vi "Test.vi"() -> ()   [LabVIEW 2012]
uses:
  Hover Button.xctl
  Button Colors.ctl
  Font Properties.ctl
panel:
  in  "Font":T1
  out "Error Out":errorcluster
  in  "Error In":errorcluster
  in  "Show Boolean Text":bool
  in  "Multiple Strings":bool
  in  "Hover Color":T2={"On Color"=16776960, "Text Color"=0, "Off Color"=16776960}
  in  "Button Color":T2={"On Color"=16860, "Text Color"=16777226, "Off Color"=16860}
  in  "Boolean Text":string[](array[string])=["Off", "Off"]
  in  "stop":bool
  in  "Hover Button":bool(xcontrol)
  # "This is a test vi for the Hover Button Xcontrol.  You should be able\nto click the right button selection menu to change the Hover Button\nProperties.  The controls on the right of the Hover Button show the\nuse of the property nodes defined for the Hover Button."
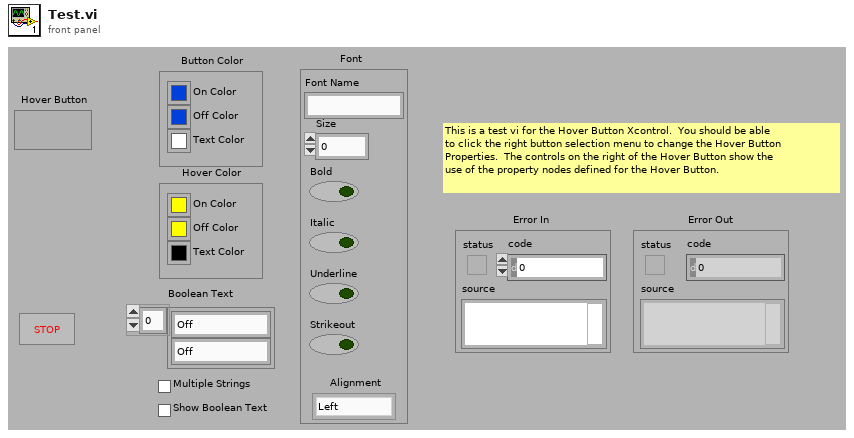
[diagram p1: front panel]
types:
  T1 = typedef "Hover Button.xctl/Font Properties.ctl" = cluster{"Font Name":string, "Size":u32, "Bold":bool, "Italic":bool, "Underline":bool, "Strikeout":bool, "Alignment":enum16{"Left", "Center", "Right"}}
  T2 = typedef "Hover Button.xctl/Button Colors.ctl" = cluster{"On Color":u32, "Text Color":u32, "Off Color":u32}
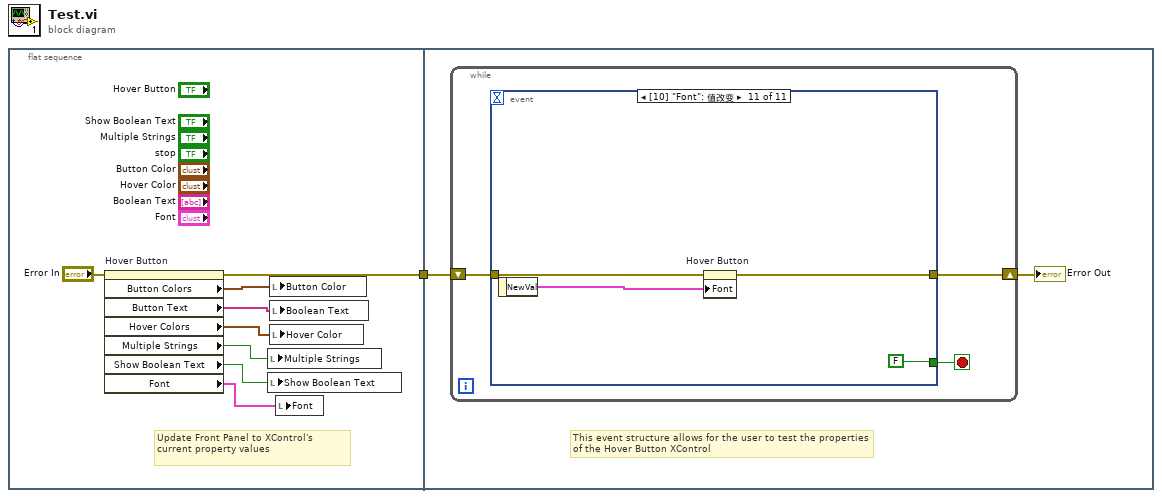
[diagram p0: block diagram]
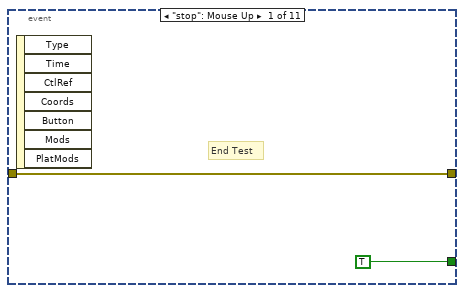
[diagram p2: hidden frame]
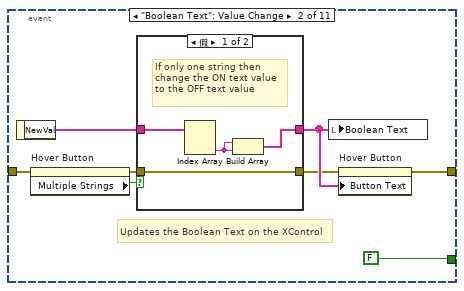
[diagram p3: hidden frame]
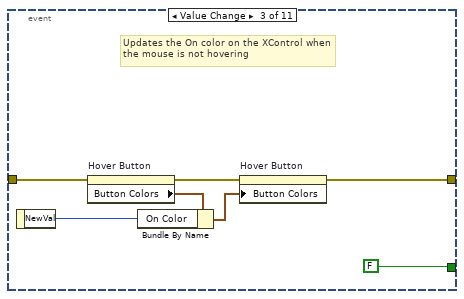
[diagram p5: hidden frame]
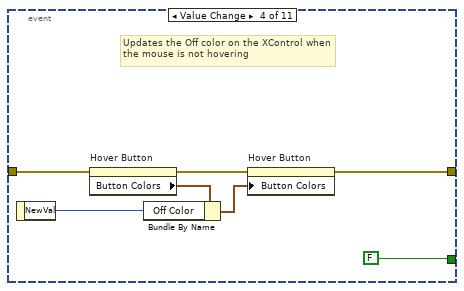
[diagram p6: hidden frame]
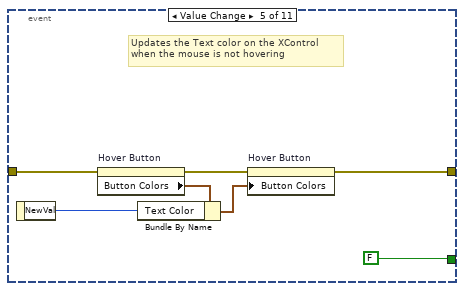
[diagram p7: hidden frame]
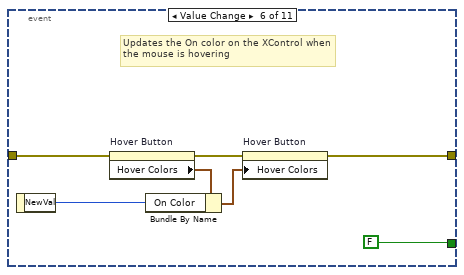
[diagram p8: hidden frame]
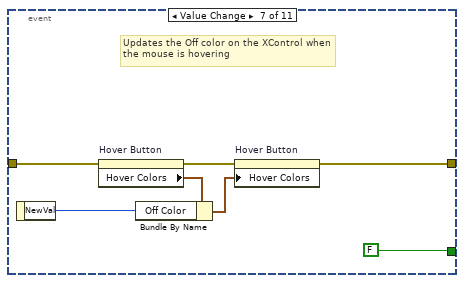
[diagram p9: hidden frame]
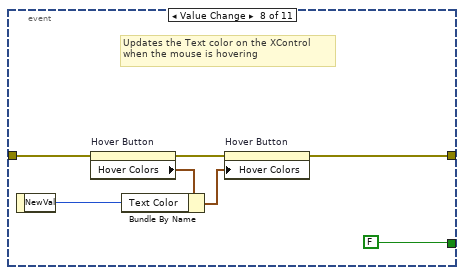
[diagram p10: hidden frame]
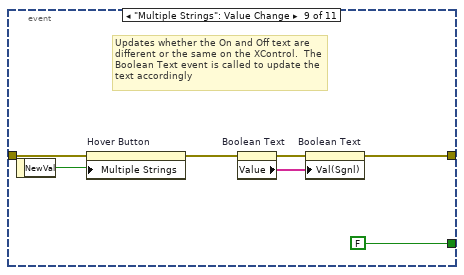
[diagram p11: hidden frame]
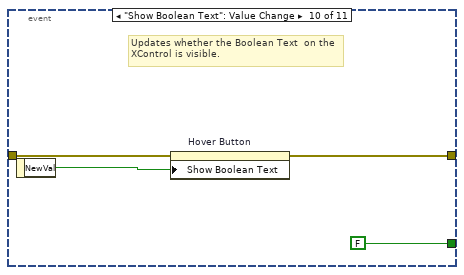
[diagram p12: hidden frame]
diagram:
  n1 = flat-sequence {
    tunnel: [w3] -> w1
    tunnel: w1 -> [w11]
    frame #0 {
      # "Update Front Panel to XControl's\ncurrent property values"
      n2 = property on="Hover Button" class="Hover Button (严格)"(error in="Error In") -> (error out=w3:errorcluster, "Button Colors"=w9:T2, "Button Text"=w7:string[], "Hover Colors"=w8:T2, "Multiple Strings"=w6:bool, "Show Boolean Text"=w5:bool, "Font"=w2:T1)  [unwired: 1 in, 1 out]
      n3 = local write "Multiple Strings"(w6) -> ()
      n4 = local write "Show Boolean Text"(w5) -> ()
      n5 = local write "Button Color"(w9) -> ()
      n6 = local write "Boolean Text"(w7) -> ()
      n7 = local write "Hover Color"(w8) -> ()
      n8 = local write "Font"(w2) -> ()
    }
    frame #1 {
      # "This event structure allows for the user to test the properties\nof the Hover Button XControl"
      n9 = while {
        shift-right: [w12] -> w10
        shift-left: w11 -> [w13]
        stop <- w14 stop-if-true
        n10 = event shown="[10] \"Font\": 值改变" {
          selector: _ -> [_ _ _ _ _ _ _ _ _ _ _]
          dyn-events: _ -> [_ _ _ _ _ _ _ _ _ _ _]
          timeout: _ -> [_ _ _ _ _ _ _ _ _ _ _]
          tunnel: [TRUE FALSE FALSE FALSE FALSE FALSE FALSE FALSE FALSE FALSE FALSE] -> w14
          tunnel: w13 -> [w15 w20 w33 w40 w47 w54 w61 w68 w74 w81 w85]
          tunnel: [w15 w18 w31 w38 w45 w52 w59 w66 w73 w80 w84] -> w12
          event "stop": Mouse Up {
            # "End Test"
            n11 = event-data() -> ()  [unwired: 1 in, 7 out]
          }
          event "Boolean Text": Value Change {
            # "Updates the Boolean Text on the XControl"
            n12 = event-data() -> ("NewVal"=w23:string[])  [unwired: 1 in]
            n13 = property on="Hover Button" class="Hover Button (严格)"(error in=w20) -> (error out=w19:errorcluster, "Multiple Strings"=w22:bool)  [unwired: 1 in, 1 out]
            n14 = case shown="假" w22 {
              tunnel: w23 -> [w28 w30]
              tunnel: [w27 w30] -> w21
              tunnel: w19 -> [w25 w29]
              tunnel: [w25 w29] -> w17
              frame False {
                # "If only one string then change the ON text value to the OFF text value"
                n15 = Index Array(array=w28) -> (element #2=w26:string)  [unwired: 2 in, 1 out]
                n16 = Build Array(w26, w26) -> (w27:string[])
              }
              frame True {
                # "If multiple strings then do nothing"
              }
            }
            n17 = local write "Boolean Text"(w21) -> ()
            n18 = property on="Hover Button" class="Hover Button (严格)"(error in=w17, "Button Text"=w21) -> (error out=w18:errorcluster)  [unwired: 1 in, 1 out]
          }
          event Value Change {
            # "Updates the On color on the XControl when the mouse is not hovering"
            n19 = event-data() -> ("NewVal"=w36:u32)  [unwired: 1 in]
            n20 = property on="Hover Button" class="Hover Button (严格)"(error in=w33) -> (error out=w32:errorcluster, "Button Colors"=w37:T2)  [unwired: 1 in, 1 out]
            n21 = Bundle By Name(cluster=w37, "On Color"=w36) -> (w35:T2)
            n22 = property on="Hover Button" class="Hover Button (严格)"(error in=w32, "Button Colors"=w35) -> (error out=w31:errorcluster)  [unwired: 1 in, 1 out]
          }
          event Value Change {
            # "Updates the Off color on the XControl when the mouse is not hovering"
            n23 = event-data() -> ("NewVal"=w43:u32)  [unwired: 1 in]
            n24 = property on="Hover Button" class="Hover Button (严格)"(error in=w40) -> (error out=w39:errorcluster, "Button Colors"=w44:T2)  [unwired: 1 in, 1 out]
            n25 = Bundle By Name(cluster=w44, "Off Color"=w43) -> (w42:T2)
            n26 = property on="Hover Button" class="Hover Button (严格)"(error in=w39, "Button Colors"=w42) -> (error out=w38:errorcluster)  [unwired: 1 in, 1 out]
          }
          event Value Change {
            # "Updates the Text color on the XControl when the mouse is not hovering"
            n27 = event-data() -> ("NewVal"=w50:u32)  [unwired: 1 in]
            n28 = property on="Hover Button" class="Hover Button (严格)"(error in=w47) -> (error out=w46:errorcluster, "Button Colors"=w51:T2)  [unwired: 1 in, 1 out]
            n29 = Bundle By Name(cluster=w51, "Text Color"=w50) -> (w49:T2)
            n30 = property on="Hover Button" class="Hover Button (严格)"(error in=w46, "Button Colors"=w49) -> (error out=w45:errorcluster)  [unwired: 1 in, 1 out]
          }
          event Value Change {
            # "Updates the On color on the XControl when the mouse is hovering"
            n31 = event-data() -> ("NewVal"=w57:u32)  [unwired: 1 in]
            n32 = property on="Hover Button" class="Hover Button (严格)"(error in=w54) -> (error out=w53:errorcluster, "Hover Colors"=w58:T2)  [unwired: 1 in, 1 out]
            n33 = Bundle By Name(cluster=w58, "On Color"=w57) -> (w56:T2)
            n34 = property on="Hover Button" class="Hover Button (严格)"(error in=w53, "Hover Colors"=w56) -> (error out=w52:errorcluster)  [unwired: 1 in, 1 out]
          }
          event Value Change {
            # "Updates the Off color on the XControl when the mouse is hovering"
            n35 = event-data() -> ("NewVal"=w64:u32)  [unwired: 1 in]
            n36 = property on="Hover Button" class="Hover Button (严格)"(error in=w61) -> (error out=w60:errorcluster, "Hover Colors"=w65:T2)  [unwired: 1 in, 1 out]
            n37 = Bundle By Name(cluster=w65, "Off Color"=w64) -> (w63:T2)
            n38 = property on="Hover Button" class="Hover Button (严格)"(error in=w60, "Hover Colors"=w63) -> (error out=w59:errorcluster)  [unwired: 1 in, 1 out]
          }
          event Value Change {
            # "Updates the Text color on the XControl when the mouse is hovering"
            n39 = event-data() -> ("NewVal"=w71:u32)  [unwired: 1 in]
            n40 = property on="Hover Button" class="Hover Button (严格)"(error in=w68) -> (error out=w67:errorcluster, "Hover Colors"=w72:T2)  [unwired: 1 in, 1 out]
            n41 = Bundle By Name(cluster=w72, "Text Color"=w71) -> (w70:T2)
            n42 = property on="Hover Button" class="Hover Button (严格)"(error in=w67, "Hover Colors"=w70) -> (error out=w66:errorcluster)  [unwired: 1 in, 1 out]
          }
          event "Multiple Strings": Value Change {
            # "Updates whether the On and Off text are different or the same on the XControl.  The Boolean Text event is called to update the text accordingly"
            n43 = event-data() -> ("NewVal"=w79:bool)  [unwired: 1 in]
            n44 = property on="Hover Button" class="Hover Button (严格)"(error in=w74, "Multiple Strings"=w79) -> (error out=w77:errorcluster)  [unwired: 1 in, 1 out]
            n45 = property on="Boolean Text" class="Arr (严格)"(error in=w77) -> (error out=w76:errorcluster, "Value"=w75:string[])  [unwired: 1 in, 1 out]
            n46 = property on="Boolean Text" class="Arr (严格)"(error in=w76, "Val(Sgnl)"=w75) -> (error out=w73:errorcluster)  [unwired: 1 in, 1 out]
          }
          event "Show Boolean Text": Value Change {
            # "Updates whether the Boolean Text  on the XControl is visible."
            n47 = event-data() -> ("NewVal"=w83:bool)  [unwired: 1 in]
            n48 = property on="Hover Button" class="Hover Button (严格)"(error in=w81, "Show Boolean Text"=w83) -> (error out=w80:errorcluster)  [unwired: 1 in, 1 out]
          }
          event Value Change {
            n49 = event-data() -> ("NewVal"=w86:T1)  [unwired: 1 in]
            n50 = property on="Hover Button" class="Hover Button (严格)"(error in=w85, "Font"=w86) -> (error out=w84:errorcluster)  [unwired: 1 in, 1 out]
          }
        }
      }
      "Error Out" <- w10
    }
  }
